vi "Error Check Missing Variant Data.vi"(8 "error in (no error)":errorcluster, 11 "Found?":bool) -> (0 "error out":errorcluster)   [LabVIEW 2020, in "Internal Comm Classes.lvlib" / "WPL Comm.lvclass"]
uses:
  WPL Comm.lvclass
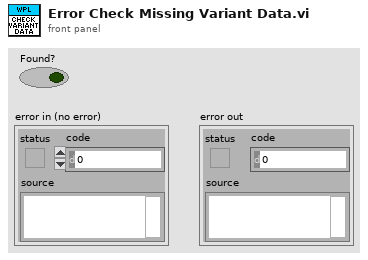
[diagram p1: front panel]
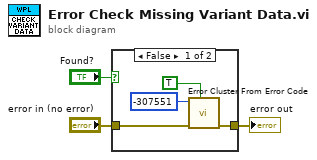
[diagram p0: block diagram]
diagram:
  n1 = case shown="False" "Found?" {
    tunnel: "error in (no error)" -> [w7 w8]
    tunnel: [w6 w8] -> w3
    frame False {
      n2 = call <vilib>:"Error Cluster From Error Code.vi"("show call chain? (False)"=TRUE, "error in (no error)"=w7, "error code (0)"=-307551) -> ("error out"=w6:errorcluster)  [unwired: 6 in]
    }
    frame True {
    }
  }
  "error out" <- w3
